vi "Check for Kill.vi"(0 "Bd ID In":T4, 1 "Kill All":bool, 2 "Stop Type":u16(ring) items=["Decelerate", "Halt", "Kill"], 5 "Controls":T1={"Axis 1"={"Axis"=1, "Enable"=FALSE, "Start"=FALSE, "Home"=FALSE, "Stop Type"=0, "Kill"=FALSE}, "Axis 2"={"Axis"=1, "Enable"=FALSE, "Start"=FALSE, "Home"=FALSE, "Stop Type"=0, "Kill"=FALSE}, "Axis 3"={"Axis"=1, "Enable"=FALSE, "Start"=FALSE, "Home"=FALSE, "Stop Type"=0, "Kill"=FALSE}, "Axis 4"={"Axis"=1, "Enable"=FALSE, "Start"=FALSE, "Home"=FALSE, "Stop Type"=0, "Kill"=FALSE}, "Axis 5"={"Axis"=1, "Enable"=FALSE, "Start"=FALSE, "Home"=FALSE, "Stop Type"=0, "Kill"=FALSE}, "Axis 6"={"Axis"=1, "Enable"=FALSE, "Start"=FALSE, "Home"=FALSE, "Stop Type"=0, "Kill"=FALSE}} {"Axis 6"."Stop Type" items=["Decelerate", "Halt", "Kill"]; "Axis 6"."Axis" items=["Axis 1"=1, "Axis 2"=2, "Axis 3"=3, "Axis 4"=4, "Axis 5"=5, "Axis 6"=6, "Axis 7"=7, "Axis 8"=8]; "Axis 5"."Stop Type" items=["Decelerate", "Halt", "Kill"]; "Axis 5"."Axis" items=["Axis 1"=1, "Axis 2"=2, "Axis 3"=3, "Axis 4"=4, "Axis 5"=5, "Axis 6"=6, "Axis 7"=7, "Axis 8"=8]; "Axis 4"."Stop Type" items=["Decelerate", "Halt", "Kill"]; "Axis 4"."Axis" items=["Axis 1"=1, "Axis 2"=2, "Axis 3"=3, "Axis 4"=4, "Axis 5"=5, "Axis 6"=6, "Axis 7"=7, "Axis 8"=8]; "Axis 3"."Stop Type" items=["Decelerate", "Halt", "Kill"]; "Axis 3"."Axis" items=["Axis 1"=1, "Axis 2"=2, "Axis 3"=3, "Axis 4"=4, "Axis 5"=5, "Axis 6"=6, "Axis 7"=7, "Axis 8"=8]; "Axis 2"."Stop Type" items=["Decelerate", "Halt", "Kill"]; "Axis 2"."Axis" items=["Axis 1"=1, "Axis 2"=2, "Axis 3"=3, "Axis 4"=4, "Axis 5"=5, "Axis 6"=6, "Axis 7"=7, "Axis 8"=8]; "Axis 1"."Stop Type" items=["Decelerate", "Halt", "Kill"]; "Axis 1"."Axis" items=["Axis 1"=1, "Axis 2"=2, "Axis 3"=3, "Axis 4"=4, "Axis 5"=5, "Axis 6"=6, "Axis 7"=7, "Axis 8"=8]}, 11 "error in":errorcluster) -> (4 "Bd ID Out":T4, 15 "error out":errorcluster)   [LabVIEW 2010]
doc: "Written specifically for the MultiAxisMove VI. Polls the 'Controls' cluster for a 'Kill' or 'Kill All' signal. If 'Kill All' is true, the Kill Axes VI is called for all axes in parallel using the given 'Stop Type'. Otherwise, function checks for a true 'Kill' condition on each axes in parallel and calls the Kill Axes subVI accordingly, using the given 'Stop Type'."
uses:
  Typedefs/AxisSpaceControls_ClusterofAxisControls.ctl
  Typedefs/AxisControls_cluster.ctl
  <vilib>/Motion/FlexMotion/CustomControls/CustomControls.llb/Axis To Control.flx
  <vilib>/Motion/FlexMotion/CustomControls/CustomControls.llb/Axis # (8 axes).flx
  <vilib>/Motion/FlexMotion/FunctionsVIs/StartStopMotion.llb/Stop Motion (8 axes).flx
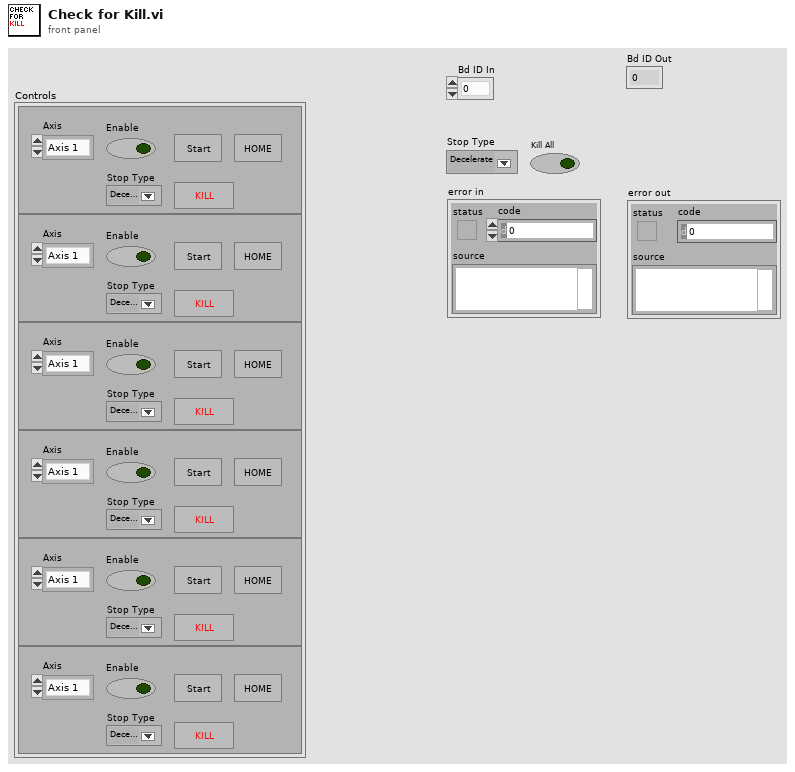
[diagram p1: front panel]
types:
  T1 = typedef "AxisSpaceControls_ClusterofAxisControls.ctl" = cluster{"Axis 1":T2, "Axis 2":T2, "Axis 3":T2, "Axis 4":T2, "Axis 5":T2, "Axis 6":T2}
  T2 = typedef "AxisControls_cluster.ctl" = cluster{"Axis":T3, "Enable":bool, "Start":bool, "Home":bool, "Stop Type":u16, "Kill":bool}
  T3 = typedef "Axis To Control.flx" = u16
  T4 = typedef "Bd Id Out" = u8
  T5 = typedef "Axis # (8 axes).flx" = cluster{"1":bool, "2":bool, "3":bool, "4":bool, "5":bool, "6":bool, "7":bool, "8":bool}
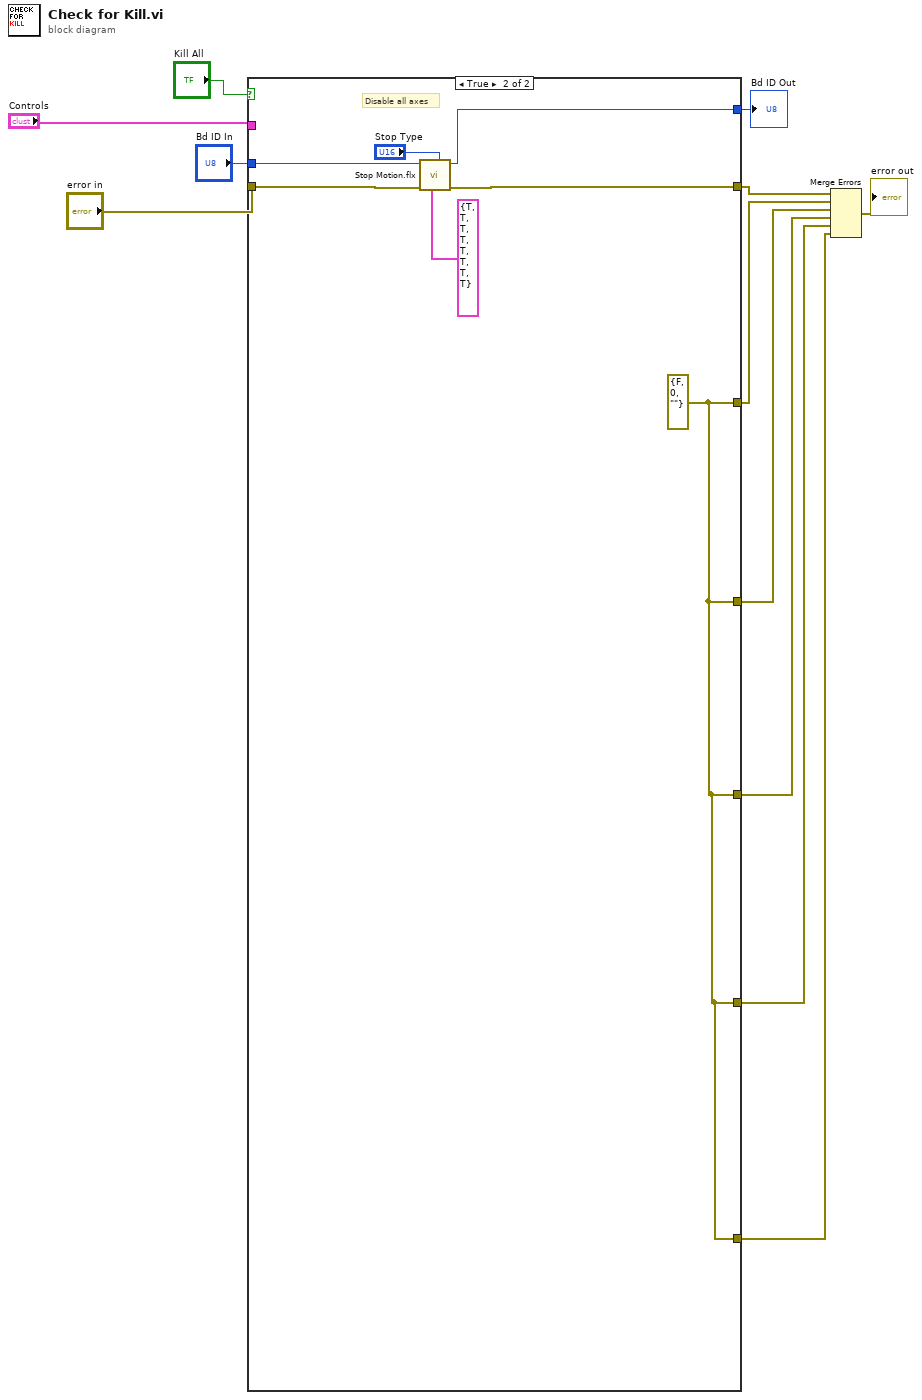
[diagram p0: block diagram]
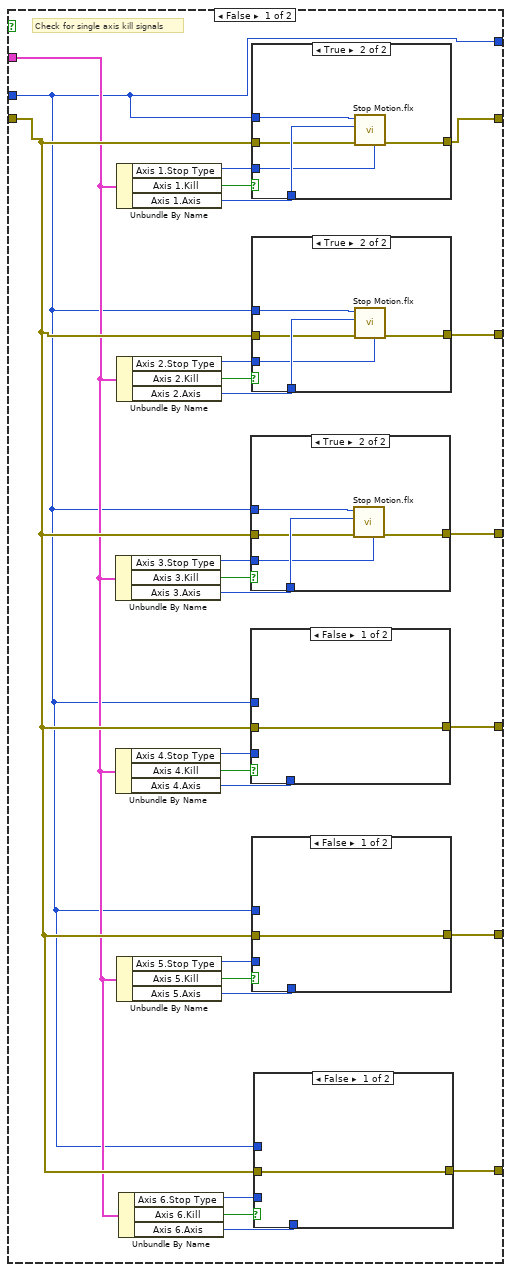
[diagram p2: hidden frame]
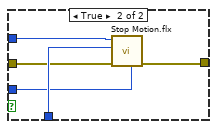
[diagram p3: hidden frame]
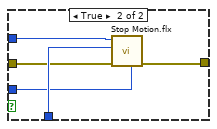
[diagram p4: hidden frame]
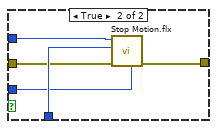
[diagram p5: hidden frame]
diagram:
  n1 = case shown="True" "Kill All" {
    tunnel: "Bd ID In" -> [w15 w82]
    tunnel: [w36 w81] -> w9
    tunnel: "error in" -> [w17 w80]
    tunnel: [w32 w76] -> w8
    tunnel: "Controls" -> [w16 _]
    tunnel: [w15 w77] -> w6
    tunnel: [w25 w76] -> w4
    tunnel: [w24 w76] -> w3
    tunnel: [w14 w76] -> w2
    tunnel: [w13 w76] -> w1
    frame False {
      # "Check for single axis kill signals"
      n2 = Unbundle By Name(w16) -> ("Axis 3.Stop Type"=w29:u16, "Axis 3.Kill"=w30:bool, "Axis 3.Axis"=w31:T3)
      n3 = Unbundle By Name(w16) -> ("Axis 4.Stop Type"=w26:u16, "Axis 4.Kill"=w27:bool, "Axis 4.Axis"=w28:T3)
      n4 = Unbundle By Name(w16) -> ("Axis 1.Stop Type"=w37:u16, "Axis 1.Kill"=w38:bool, "Axis 1.Axis"=w39:T3)
      n5 = Unbundle By Name(w16) -> ("Axis 2.Stop Type"=w33:u16, "Axis 2.Kill"=w34:bool, "Axis 2.Axis"=w35:T3)
      n6 = Unbundle By Name(w16) -> ("Axis 5.Stop Type"=w21:u16, "Axis 5.Kill"=w22:bool, "Axis 5.Axis"=w23:T3)
      n7 = Unbundle By Name(w16) -> ("Axis 6.Stop Type"=w18:u16, "Axis 6.Kill"=w19:bool, "Axis 6.Axis"=w20:T3)
      n8 = case shown="True" w30 {
        tunnel: [w58 w63] -> w25
        tunnel: w31 -> [_ w62]
        tunnel: w29 -> [_ w61]
        tunnel: w17 -> [w58 w60]
        tunnel: w15 -> [_ w59]
        frame False {
        }
        frame True {
          n9 = call-poly <vilib>:"Stop Motion.flx"("Stop Type (Decel)"=w61, "error in (no error)"=w60, "Axis or Vector Space"=w62, "Board ID"=w59) -> ("error out"=w63:errorcluster)  [unwired: 3 in, 2 out]
        }
      }
      n10 = case shown="False" w27 {
        tunnel: [w52 w57] -> w24
        tunnel: w28 -> [_ w56]
        tunnel: w26 -> [_ w55]
        tunnel: w17 -> [w52 w54]
        tunnel: w15 -> [_ w53]
        frame False {
        }
        frame True {
          n11 = call-poly <vilib>:"Stop Motion.flx"("Stop Type (Decel)"=w55, "error in (no error)"=w54, "Axis or Vector Space"=w56, "Board ID"=w53) -> ("error out"=w57:errorcluster)  [unwired: 3 in, 2 out]
        }
      }
      n12 = case shown="True" w38 {
        tunnel: [w70 w75] -> w36
        tunnel: w39 -> [_ w74]
        tunnel: w37 -> [_ w73]
        tunnel: w17 -> [w70 w72]
        tunnel: w15 -> [_ w71]
        frame False {
        }
        frame True {
          n13 = call-poly <vilib>:"Stop Motion.flx"("Stop Type (Decel)"=w73, "error in (no error)"=w72, "Axis or Vector Space"=w74, "Board ID"=w71) -> ("error out"=w75:errorcluster)  [unwired: 3 in, 2 out]
        }
      }
      n14 = case shown="True" w34 {
        tunnel: [w64 w69] -> w32
        tunnel: w35 -> [_ w68]
        tunnel: w33 -> [_ w67]
        tunnel: w17 -> [w64 w66]
        tunnel: w15 -> [_ w65]
        frame False {
        }
        frame True {
          n15 = call-poly <vilib>:"Stop Motion.flx"("Stop Type (Decel)"=w67, "error in (no error)"=w66, "Axis or Vector Space"=w68, "Board ID"=w65) -> ("error out"=w69:errorcluster)  [unwired: 3 in, 2 out]
        }
      }
      n16 = case shown="False" w22 {
        tunnel: [w46 w51] -> w14
        tunnel: w23 -> [_ w50]
        tunnel: w21 -> [_ w49]
        tunnel: w17 -> [w46 w48]
        tunnel: w15 -> [_ w47]
        frame False {
        }
        frame True {
          n17 = call-poly <vilib>:"Stop Motion.flx"("Stop Type (Decel)"=w49, "error in (no error)"=w48, "Axis or Vector Space"=w50, "Board ID"=w47) -> ("error out"=w51:errorcluster)  [unwired: 3 in, 2 out]
        }
      }
      n18 = case shown="False" w19 {
        tunnel: [w40 w45] -> w13
        tunnel: w20 -> [_ w44]
        tunnel: w18 -> [_ w43]
        tunnel: w17 -> [w40 w42]
        tunnel: w15 -> [_ w41]
        frame False {
        }
        frame True {
          n19 = call-poly <vilib>:"Stop Motion.flx"("Stop Type (Decel)"=w43, "error in (no error)"=w42, "Axis or Vector Space"=w44, "Board ID"=w41) -> ("error out"=w45:errorcluster)  [unwired: 3 in, 2 out]
        }
      }
    }
    frame True {
      w76 = errorcluster {"status"=FALSE, "code"=0, "source"=""} ("error out")
      # "Disable all axes"
      n20 = call-poly <vilib>:"Stop Motion.flx"("Stop Type (Decel)"="Stop Type", "Axis/VS Map (Disabled)"=T5 {"1"=TRUE, "2"=TRUE, "3"=TRUE, "4"=TRUE, "5"=TRUE, "6"=TRUE, "7"=TRUE, "8"=TRUE}, "error in (no error)"=w80, "Board ID"=w82) -> ("error out"=w81:errorcluster, "Bd ID Out"=w77:T4)  [unwired: 3 in, 1 out]
    }
  }
  "Bd ID Out" <- w6
  n21 = Merge Errors(w9, w8, w4, w3, w2, w1) -> (→"error out":errorcluster)
